vi "Формирователь флагов.vi"(5 "Type":bool, 6 "s1":bool, 7 "R":T1) -> (0 "Type":bool, 1 "ZF":bool, 2 "Err":bool, 3 "CF":bool)   [LabVIEW 2013]
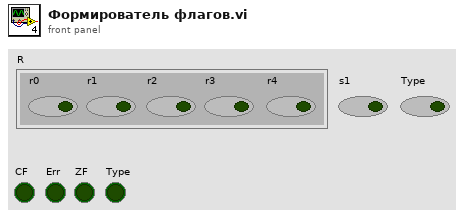
[diagram p1: front panel]
types:
  T1 = cluster{"r0":bool, "r1":bool, "r2":bool, "r3":bool, "r4":bool}
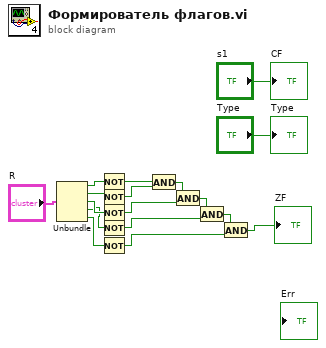
[diagram p0: block diagram]
diagram:
  n1 = Unbundle("R") -> ("r0"=w14:bool, "r1"=w13:bool, "r2"=w12:bool, "r3"=w11:bool, "r4"=w10:bool)
  n2 = Not(x=w14) -> (.not. x?=w9:bool)
  n3 = Not(x=w13) -> (.not. x?=w8:bool)
  n4 = Not(x=w12) -> (.not. x?=w7:bool)
  n5 = Not(x=w11) -> (.not. x?=w6:bool)
  n6 = Not(x=w10) -> (.not. x?=w5:bool)
  n7 = And(x=w9, y=w8) -> (x .and. y?=w4:bool)
  n8 = And(x=w4, y=w7) -> (x .and. y?=w3:bool)
  n9 = And(x=w3, y=w6) -> (x .and. y?=w2:bool)
  n10 = And(x=w2, y=w5) -> (x .and. y?=→"ZF":bool)
  "CF" <- "s1"
  "Type" <- "Type"
